vi "Rec Save Recordset To File (R).vi"(5 "overwrite? (F)":bool, 6 "error in (no error)":errorcluster, 7 "save format (XML)":T1=enum."XML", 8 "file name":path, 9 "recordset reference":T2) -> (0 "error out":errorcluster, 3 "recordset reference out":T2)   [LabVIEW 2013, in "NI_Database_API_64.lvlib"]
doc: "Saves the recordset identified by the <B>recordset reference</B> to either an XML or ADTG file. The ADTG file format is a proprietary format that only the LabVIEW Database Connectivity Toolkit can interpret. The ADTG format results in a smaller file than the XML format. You can reload both formats into LabVIEW using the DB Tools Load Recordset From File VI.\n\nWire data to the reference input to determine the polymorphic instance to use or manually select the instance."
uses:
  NI_Database_API_64.lvlib
  Rec ObjectReference.ctl
  Rec Save Format.ctl
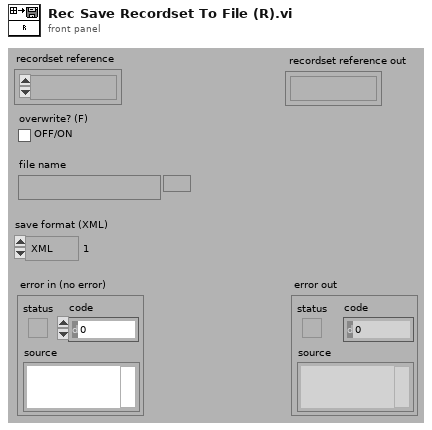
[diagram p1: front panel]
types:
  T1 = typedef "NI_Database_API_64.lvlib/Rec Save Format.ctl" = enum16{"ADTG", "XML"}
  T2 = typedef "NI_Database_API_64.lvlib/Rec ObjectReference.ctl" = refnum<k1>
  T3 = typedef "NI_Database_API_64.lvlib/Rec DataMembers.ctl" = cluster{"ADODB._Recordset":refnum<k7>, "Connection":T4}
  T4 = typedef "NI_Database_API_64.lvlib/Conn ObjectReference.ctl" = refnum<k1>
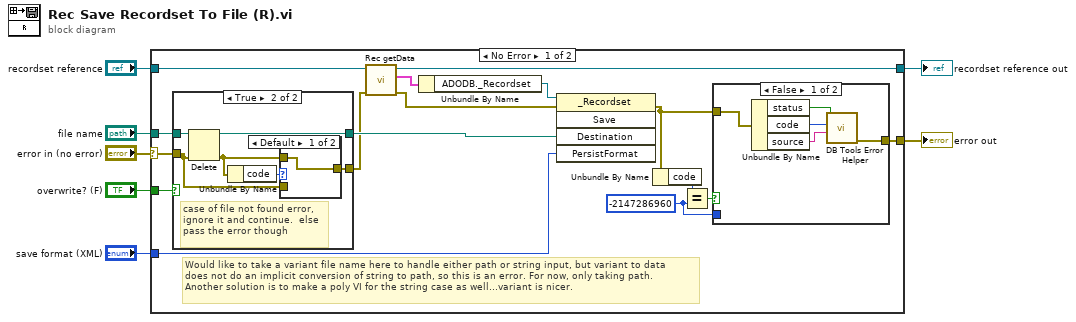
[diagram p0: block diagram]
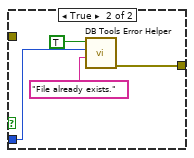
[diagram p2: hidden frame]
diagram:
  n1 = case shown="No Error" "error in (no error)" {
    selector: "error in (no error)" -> [w10 w44]
    tunnel: "overwrite? (F)" -> [w23 _]
    tunnel: "file name" -> [w22 _]
    tunnel: "save format (XML)" -> [w20 _]
    tunnel: "recordset reference" -> [w18 w43]
    tunnel: [w15 w43] -> w3
    tunnel: [w9 w44] -> w2
    frame No Error {
      w11 = -2147286960 ("code")
      # "Would like to take a variant file name here to handle either path or string input, but variant to data\ndoes not do an implicit conversion of string to path, so this is an error. For now, only taking path.\nAnother solution is to make a poly VI for the string case as well...variant is nicer."
      n2 = case shown="True" w23 {
        tunnel: w10 -> [w33 w36]
        tunnel: w22 -> [w34 w40]
        tunnel: [w34 w39] -> w21
        tunnel: [w33 w35] -> w8
        frame False {
        }
        frame True {
          # "case of file not found error,\nignore it and continue.  else\npass the error though"
          n3 = Delete(path (use dialog)=w40, error in=w36) -> (deleted path=w39:path, error out=w37:errorcluster)  [unwired: 4 out]
          n4 = Unbundle By Name(w37) -> ("code"=w38:i32)
          n5 = case shown="Default" w38 {
            tunnel: w37 -> [w41 _]
            tunnel: w36 -> [_ w42]
            tunnel: [w41 w42] -> w35
            frame Default {
            }
            frame 7 {
            }
          }
        }
      }
      n6 = call "Rec getData.vi"("error in (no error)"=w8, "recordset reference"=w18) -> ("error out"=w17:errorcluster, "data"=w19:T3, "recordset reference out"=w15:T2)  [unwired: 3 out]
      n7 = Unbundle By Name(w19) -> ("ADODB._Recordset"=w16:refnum<k7>)
      n8 = invoke class="_Recordset" method="Save"(reference=w16, error in=w17, "Destination"=w21, "PersistFormat"=w20) -> (error out=w14:errorcluster)  [unwired: 1 in, 4 out]
      n9 = Unbundle By Name(w14) -> ("code"=w13:i32)
      n10 = Equal?(x=w13, y=w11) -> (x = y?=w12:bool)
      n11 = case shown="False" w12 {
        tunnel: w14 -> [w28 _]
        tunnel: w11 -> [_ w31]
        tunnel: [w24 w29] -> w9
        frame False {
          n12 = Unbundle By Name(w28) -> ("status"=w25:bool, "code"=w26:i32, "source"=w27:string)
          n13 = call "DB Tools Error Helper.vi"("source"=w27, "code"=w26, "status"=w25) -> ("error out"=w24:errorcluster)  [unwired: 1 in, 7 out]
        }
        frame True {
          n14 = call "DB Tools Error Helper.vi"("source"="File already exists.", "code"=w31, "status"=TRUE) -> ("error out"=w29:errorcluster)  [unwired: 1 in, 7 out]
        }
      }
    }
    frame Error {
    }
  }
  "recordset reference out" <- w3
  "error out" <- w2
